vi "Init.vi"(7 "Name":string, 8 "error in":errorcluster, 9 "Values":string[](array[string]), 10 "Keynames":string[](array[string]), 11 "Section in":refnum<class "Section.lvclass">) -> (0 "error out":errorcluster, 3 "Section out":refnum<class "Section.lvclass">)   [LabVIEW 2024, in "Electronic Datasheet.lvlib" / "Section.lvclass"]
uses:
  Section.lvclass
  Value/Value.lvclass
  Keyname/Key Name.lvclass
  Section.lvclass/Section.ctl
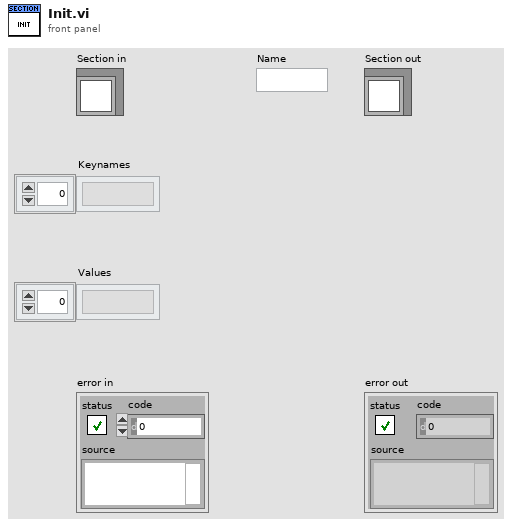
[diagram p1: front panel]
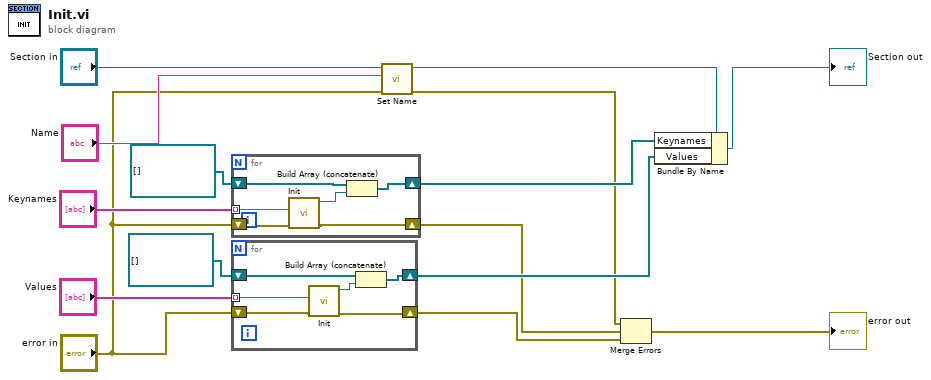
[diagram p0: block diagram]
diagram:
  n1 = for {
    tunnel: "Keynames" -> [w21] mode=indexing
    shift-right: [w18] -> w7
    shift-left: refnum<class "Key Name.lvclass">[] [] -> [w19]
    shift-right: [w16] -> w2
    shift-left: "error in" -> [w17]
    n2 = call "Init.vi"("error in"=w17, "Key Name"=w21) -> ("error out"=w16:errorcluster, "Key Name out"=w20:refnum<class "Key Name.lvclass">)  [unwired: 8 in]
    n3 = Build Array (concatenate)(w19, w20) -> (w18:refnum<class "Key Name.lvclass">[])
  }
  n4 = for {
    tunnel: "Values" -> [w27] mode=indexing
    shift-right: [w23] -> w6
    shift-left: refnum<class "Value.lvclass">[] [] -> [w26]
    shift-right: [w22] -> w11
    shift-left: "error in" -> [w24]
    n5 = call "Init.vi"("error in"=w24, "Value"=w27) -> ("error out"=w22:errorcluster, "Value out"=w25:refnum<class "Value.lvclass">)  [unwired: 8 in]
    n6 = Build Array (concatenate)(w26, w25) -> (w23:refnum<class "Value.lvclass">[])
  }
  n7 = call "Set Name.vi"("error in"="error in", "Section Name"="Name", "Object Entry in"="Section in") -> ("error out"=w3:errorcluster, "Object Entry out"=w5:refnum<class "Section.lvclass">)  [unwired: 7 in]
  n8 = Merge Errors(w3, w2, w11) -> (→"error out":errorcluster)
  n9 = Bundle By Name(cluster=w5, "Keynames"=w7, "Values"=w6) -> (→"Section out":refnum<class "Section.lvclass">)
